vi "GetInfo.vi"() -> ()   [LabVIEW 2012]
panel:
  in  "Position":i32
  in  "Message":i32
  in  "Axis to query":dbl
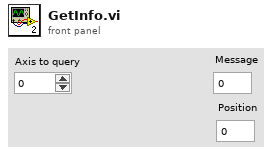
[diagram p1: front panel]
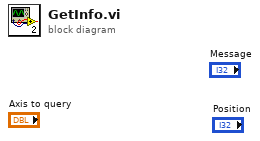
[diagram p0: block diagram]
diagram:
